vi "Evaluate magnet status.vi"(2 "PSU Status in":T8 {"Trip Current" format="%.3f"; "Trip Field" format="%.4f"; "Voltage" format="%.2f"; "Field Constant" format="%.6f"; "MID Setpoint (T)" format="%.4f"; "MID Setpoint (A)" format="%.3f"; "MAX Setpoint (T)" format="%.4f"; "MAX Setpoint (A)" format="%.3f"; "Heater Voltage" format="%.2f"; "V Limit (V)" format="%.2f"; "Ramp Rate (A/s)" format="%.3f"; "Output (A)" format="%.3f"; "Output (T)" format="%.4f"; "Persistent Current" format="%.3f"; "Persistent Field" format="%.4f"}, 3 "LSC218 sensors":T9 {"Time stamp" format="%<%H:%M:%S%2u\n%Y/%m/%d>T"}, 4 "Overall status in":T1, 5 "Magnet Constants":T7={"Switch resistant [K]"=5.0, "Switch superconducting [K]"=4.0, "First stage critical temperature [K]"=50.0, "Second stage critical temperature [K]"=5.0, "Inner magnet critical temperature [K]"=6.0, "Outer magnet critical temperature [K]"=5.0, "Field Constant [T/A]"=0.14911, "Maximum Current [A]"=107.3, "Maximum field [T]"=16.0, "Maximum source ramp [A/s]"=0.5, "Source precision [T]"=2e-05, "Ramp limits [A/s]"=[0.0506, 0.038, 0.0285, 0.0213, 0.0104], "Field limits [T]"=[3.0, 9.6, 13.3, 15.5, 16.0], "SMS"="COM3", "LSC218"="COM1"}) -> (0 "Overall status out":T1)   [LabVIEW 2022 SP3, in "Magnet module.lvlib"]
doc: "Evaluates actual overall status of the magnet module.\nResult should be send as a message to master module."
uses:
  Magnet module.lvlib
  ctl/Cryostat temperature sensors.ctl
  <instrlib>/SMS 120/Public/PSU Status.ctl
  ctl/Overall status.ctl
  ctl/SetField data.ctl
  ctl/Magnet mode public.ctl
  ctl/Actual magnet state.ctl
  ctl/Magnet mode.ctl
  ctl/RampingOutput.ctl
  ctl/Magnet config constants.ctl
  <instrlib>/SMS 120/Cryogenic Ltd SMSXXX.lvlib
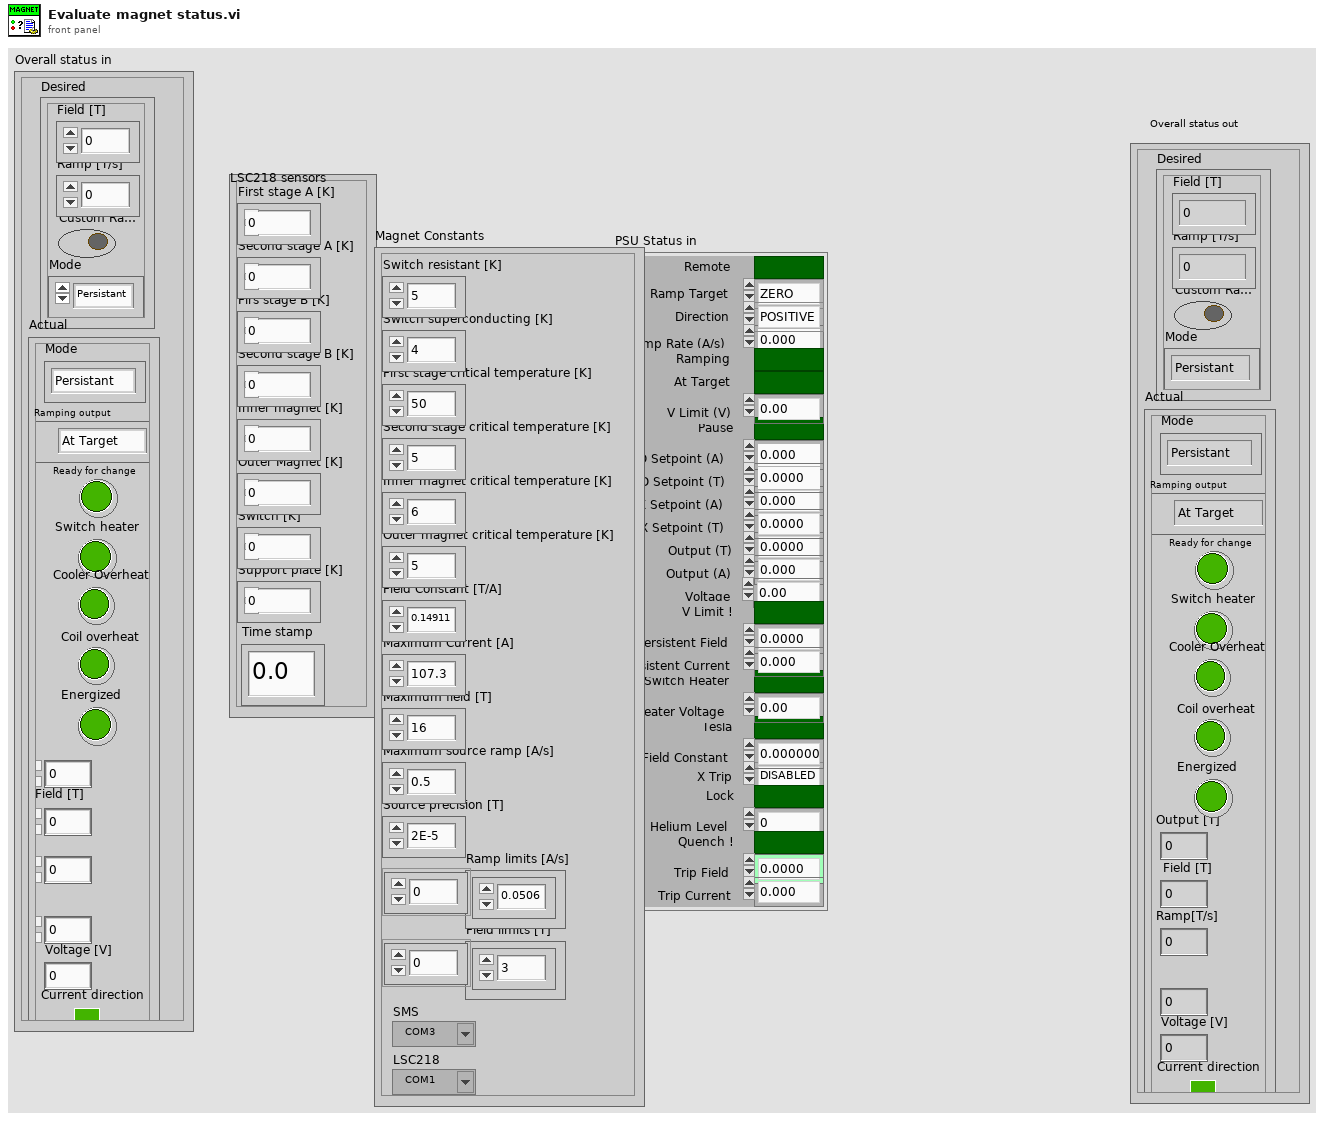
[diagram p1: front panel]
types:
  T1 = typedef "Magnet module.lvlib/Overall status.ctl" = cluster{"Desired":T2, "Actual":T4}
  T2 = typedef "Magnet module.lvlib/SetField data.ctl" = cluster{"Field [T]":dbl, "Ramp [T/s]":dbl, "Custom Ramp?":bool, "Mode":T3}
  T3 = typedef "Magnet module.lvlib/Magnet mode public.ctl" = enum16{"Persistant", "Ramping"}
  T4 = typedef "Magnet module.lvlib/Actual magnet state.ctl" = cluster{"Mode":T5, "Ramping output":T6, "Ready for change":bool, "Switch heater":bool, "Cooler Overheat":bool, "Coil overheat":bool, "Energized":bool, "Output [T]":dbl, "Field [T]":dbl, "Ramp[T/s]":dbl, "Switch\ntemperature [K]":dbl, "Voltage [V]":dbl, "Current direction":bool}
  T5 = typedef "Magnet module.lvlib/Magnet mode.ctl" = enum16{"Persistant", "Switching", "Ramping", "Quenched"}
  T6 = typedef "Magnet module.lvlib/RampingOutput.ctl" = enum16{"At Target", "Go up", "Go down"}
  T7 = typedef "Magnet module.lvlib/Magnet config constants.ctl" = cluster{"Switch resistant [K]":dbl, "Switch superconducting [K]":dbl, "First stage critical temperature [K]":dbl, "Second stage critical temperature [K]":dbl, "Inner magnet critical temperature [K]":dbl, "Outer magnet critical temperature [K]":dbl, "Field Constant [T/A]":dbl, "Maximum Current [A]":dbl, "Maximum field [T]":dbl, "Maximum source ramp [A/s]":dbl, "Source precision [T]":dbl, "Ramp limits [A/s]":dbl[], "Field limits [T]":dbl[], "SMS":refnum<visa-resource-name>, "LSC218":refnum<visa-resource-name>}
  T8 = typedef "Cryogenic Ltd SMSXXX.lvlib/PSU Status.ctl" = cluster{"Ramp Target":enum16{"ZERO", "MID", "MAX"}, "Pause":bool, "Switch Heater":bool, "Persistent Field":dbl, "Persistent Current":dbl, "Tesla":bool, "Output (T)":dbl, "Output (A)":dbl, "X Trip":enum16{"DISABLED", "ENABLED", "ACTIVE"}, "Ramp Rate (A/s)":dbl, "V Limit (V)":dbl, "Heater Voltage":dbl, "MAX Setpoint (A)":dbl, "MAX Setpoint (T)":dbl, "MID Setpoint (A)":dbl, "MID Setpoint (T)":dbl, "Lock":bool, "Field Constant":dbl, "Remote":bool, "Direction":enum16{"POSITIVE", "NEGATIVE", "OPEN", "UNIPOLAR"}, "Helium Level":u16, "Quench !":bool, "Voltage":dbl, "V Limit !":bool, "Ramping":bool, "At Target":bool, "Trip Field":dbl, "Trip Current":dbl}
  T9 = typedef "Magnet module.lvlib/Cryostat temperature sensors.ctl" = cluster{"First stage A [K]":dbl, "Second stage A [K]":dbl, "Firs stage B [K]":dbl, "Second stage B [K]":dbl, "Inner magnet [K]":dbl, "Outer Magnet [K]":dbl, "Switch [K]":dbl, "Support plate [K]":dbl, "Time stamp":dbl}
  T10 = enum16{"POSITIVE", "NEGATIVE", "OPEN", "UNIPOLAR"}
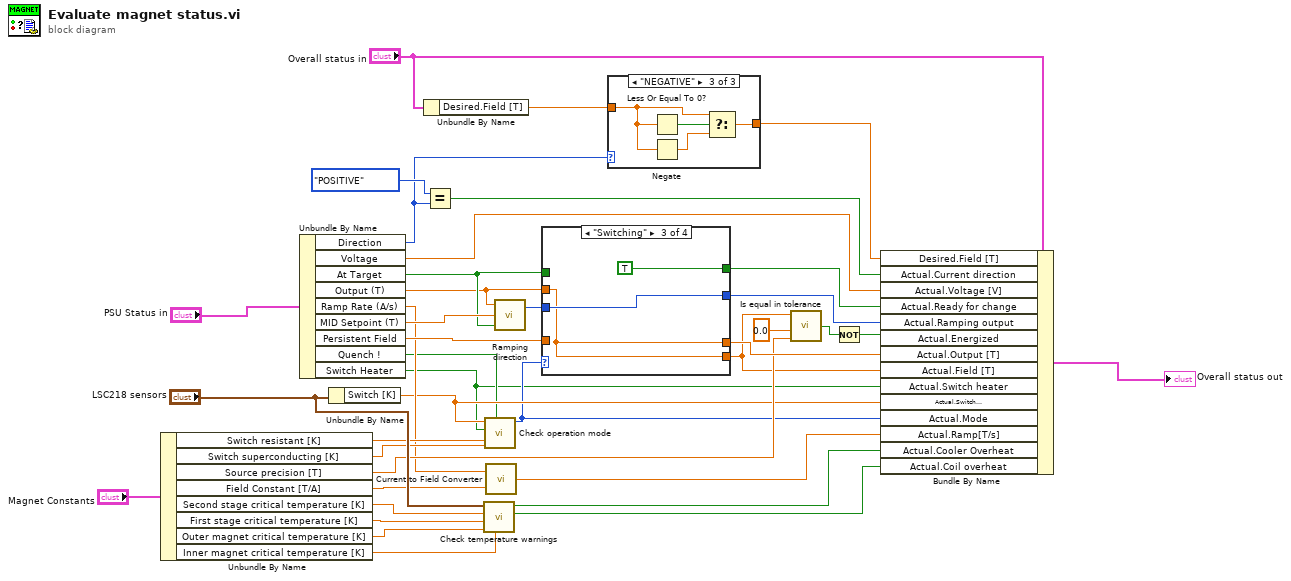
[diagram p0: block diagram]
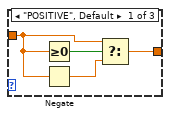
[diagram p2: hidden frame]
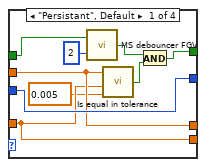
[diagram p4: hidden frame]
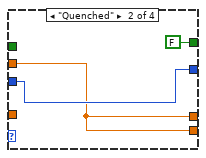
[diagram p5: hidden frame]
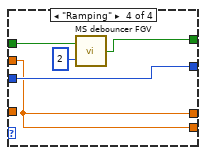
[diagram p6: hidden frame]
diagram:
  n1 = Unbundle By Name("Magnet Constants") -> ("Switch resistant [K]"=w25:dbl, "Switch superconducting [K]"=w26:dbl, "Source precision [T]"=w24:dbl, "Field Constant [T/A]"=w23:dbl, "Second stage critical temperature [K]"=w12:dbl, "First stage critical temperature [K]"=w11:dbl, "Outer magnet critical temperature [K]"=w10:dbl, "Inner magnet critical temperature [K]"=w9:dbl)
  n2 = Unbundle By Name("PSU Status in") -> ("Direction"=w2:T10, "Voltage"=w16:dbl, "At Target"=w38:bool, "Output (T)"=w37:dbl, "Ramp Rate (A/s)"=w22:dbl, "MID Setpoint (T)"=w39:dbl, "Persistent Field"=w29:dbl, "Quench !"=w18:bool, "Switch Heater"=w17:bool)
  n3 = Unbundle By Name("LSC218 sensors") -> ("Switch [K]"=w20:dbl)
  n4 = Unbundle By Name("Overall status in") -> ("Desired.Field [T]"=w4:dbl)
  n5 = Equal?(x=T10."POSITIVE" ("Direction"), y=w2) -> (x = y?=w3:bool)
  n6 = call "Check temperature warnings.vi"("Inner coil limit [K]"=w9, "Outer coil limit [K]"=w10, "1st Cryocooler limit [K]"=w11, "2nd cryocooler limit [K]"=w12, "LSC218 sensors"="LSC218 sensors") -> ("Coil Overheat"=w15:bool, "Crocooler overheat"=w8:bool)  [unwired: 4 in, 1 out]
  n7 = call "Check operation mode.vi"("Quenched?"=w18, "Switch supercond [K]"=w26, "Switch rezist [K]"=w25, "Switch Heater"=w17, "Switch actual [K]"=w20) -> ("Magnet Mode"=w19:T5)  [unwired: 6 in]
  n8 = call "Current to Field Converter.vi"("Field constant [T/A]"=w23, "Current in [A]"=w22) -> ("Field out [T]"=w21:dbl)
  n9 = call "Ramping direction.vi"("At target"=w38, "Actual targget [T]"=w39, "Actual output [T]"=w37) -> ("Ramping direction"=w30:T6)  [unwired: 1 in]
  n10 = case shown="\"Switching\"" w19 {
    tunnel: [w48 FALSE ("Is stabe") TRUE ("Ready") w59] -> w28
    tunnel: w29 -> [w45 _ _ _]
    tunnel: w37 -> [w46 w50 w52 w57]
    tunnel: w30 -> [w47 w51 w54 w58]
    tunnel: [w47 w51 w54 w58] -> w14
    tunnel: w38 -> [w40 _ _ w55]
    tunnel: [w45 w50 w52 w57] -> w13
    tunnel: [w46 w50 w52 w57] -> w34
    frame "Persistant", Default {
      n11 = call "MS debouncer FGV.vi"("Iterations"=2, "At target?"=w40) -> ("Is stabe"=w42:bool)
      n12 = call "Is equal in tolerance.vi"("Absolut tolerance"=0.005, "Reference value"=w45, "Input value"=w46) -> ("Is in range"=w44:bool)  [unwired: 1 in]
      n13 = And(x=w42, y=w44) -> (x .and. y?=w48:bool)
    }
    frame "Quenched" {
    }
    frame "Switching" {
    }
    frame "Ramping" {
      n14 = call "MS debouncer FGV.vi"("Iterations"=2, "At target?"=w55) -> ("Is stabe"=w59:bool)
    }
  }
  n15 = case shown="\"NEGATIVE\"" w2 {
    tunnel: w4 -> [w60 w64 w66]
    tunnel: [w63 w64 w65] -> w1
    frame "POSITIVE", Default {
      n16 = Greater Or Equal To 0?(x=w60) -> (x >= 0?=w62:bool)
      n17 = Negate(x=w60) -> (-x=w61:dbl)
      n18 = Select(t=w60, s=w62, f=w61) -> (s? t:f=w63:dbl)
    }
    frame "OPEN" {
    }
    frame "NEGATIVE" {
      n19 = Less Or Equal To 0?(x=w66) -> (x <= 0?=w68:bool)
      n20 = Negate(x=w66) -> (-x=w67:dbl)
      n21 = Select(t=w66, s=w68, f=w67) -> (s? t:f=w65:dbl)
    }
  }
  n22 = call "Is equal in tolerance.vi"("Absolut tolerance"=w24, "Reference value"=0.0, "Input value"=w13) -> ("Is in range"=w31:bool)  [unwired: 1 in]
  n23 = Not(x=w31) -> (.not. x?=w33:bool)
  n24 = Bundle By Name(cluster="Overall status in", "Desired.Field [T]"=w1, "Actual.Current direction"=w3, "Actual.Voltage [V]"=w16, "Actual.Ready for change"=w28, "Actual.Ramping output"=w14, "Actual.Energized"=w33, "Actual.Output [T]"=w34, "Actual.Field [T]"=w13, "Actual.Switch heater"=w17, "Actual.Switch\ntemperature [K]"=w20, "Actual.Mode"=w19, "Actual.Ramp[T/s]"=w21, "Actual.Cooler Overheat"=w8, "Actual.Coil overheat"=w15) -> (→"Overall status out":T1)
